vi "AddTemplate.vi"(8 "Error In":errorcluster, 10 "Template-VI Names":string[](array[string])) -> (0 "Error Out":errorcluster)   [LabVIEW 2016]
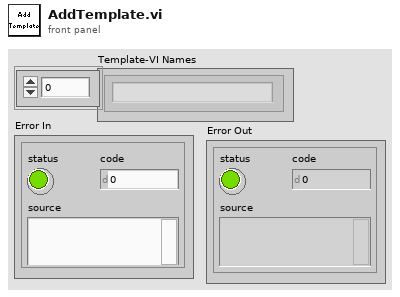
[diagram p1: front panel]
types:
  T1 = enum16{"Invalid Wire Rule", "Required", "Recommended", "Optional", "Dynamic Dispatch"}
  T2 = typedef "LVRectTypeDef.ctl" = cluster{"Left":i16, "Top":i16, "Right":i16, "Bottom":i16}
  T3 = enum16{"Invalid Wire Rule", "Required", "Recommended", "Optional", "Dynamic Dispatch"}[]
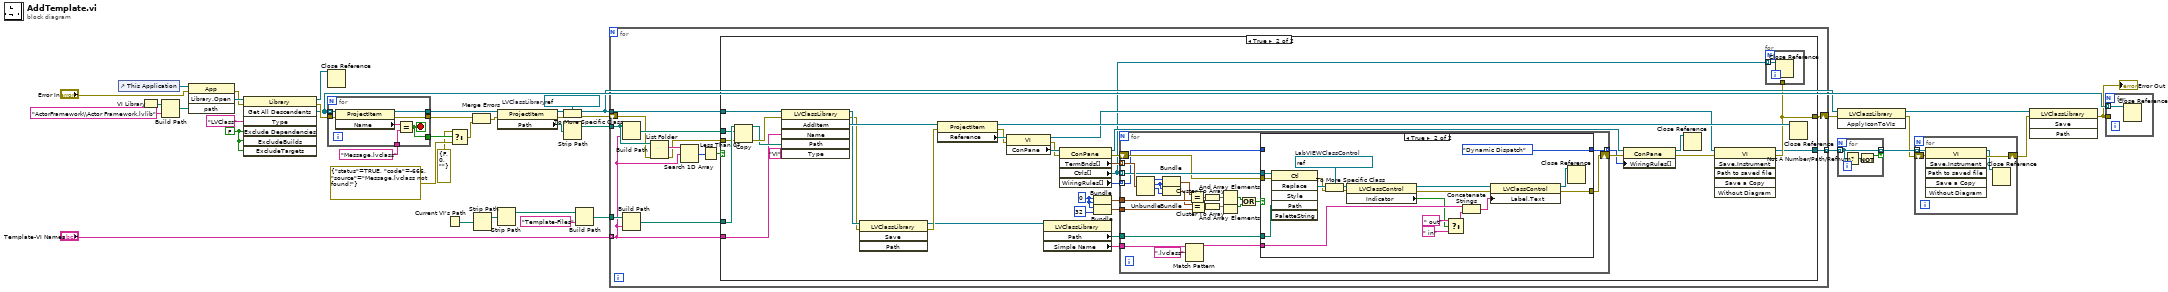
[diagram p0: block diagram]
diagram:
  w18 = refnum<vi> refnum  # LVClassLibrary
  w33 = FALSE ("ExcludeDependencies")
  n1 = control-ref of="This Application"() -> (w40:refnum<vi>)
  n2 = VI Library() -> (path=w39:path)
  n3 = Build Path(base path=w39, name or relative path="ActorFramework\\Actor Framework.lvlib") -> (appended path=w37:path)
  n4 = invoke class="App" method="Library.Open"(reference=w40, error in="Error In", "path"=w37) -> (error out=w34:errorcluster, "Open Library"=w35:refnum<vi>)  [unwired: 1 in, 2 out]
  n5 = invoke class="Library" method="Get All Descendents"(reference=w35, error in=w34, "Type"="LVClass", "Exclude Dependencies"=w33, "ExcludeBuilds"=w33, "ExcludeTargets"=w33) -> (reference out=w6:refnum<vi>, error out=w32:errorcluster, "All Descendents"=w15:refnum<vi>[])  [unwired: 1 in, 4 out]
  n6 = Close Reference(reference=w6) -> ()  [unwired: 1 in, 1 out]
  n7 = for {
    tunnel: w15 -> [w47] mode=indexing
    tunnel: "Message.lvclass" ("name") -> [w45]
    tunnel: [w44] -> w21
    tunnel: w32 -> [w43]
    tunnel: [w42] -> w26
    tunnel: [w41] -> w30
    stop <- w41 stop-if-true
    n8 = property class="ProjectItem"(reference=w47, error in=w43) -> (reference out=w44:refnum<vi>, error out=w42:errorcluster, "Name"=w46:string)
    n9 = Equal?(x=w46, y=w45) -> (x = y?=w41:bool)
  }
  n10 = Current VI's Path() -> (path=w25:path)
  n11 = Select(t=errorcluster {"status"=FALSE, "code"=0, "source"=""} ("error constant"), s=w30, f=errorcluster {"status"=TRUE, "code"=-666, "source"="Message.lvclass not found!"} ("error constant")) -> (s? t:f=w27:errorcluster)
  n12 = Merge Errors(w26, w27) -> (w20:errorcluster)
  n13 = Strip Path(path=w25) -> (stripped path=w24:path)  [unwired: 1 out]
  n14 = Strip Path(path=w24) -> (stripped path=w11:path)  [unwired: 1 out]
  n15 = property class="ProjectItem"(reference=w21, error in=w20) -> (reference out=w17:refnum<vi>, error out=w16:errorcluster, "Path"=w19:path)
  n16 = To More Specific Class(target class=w18, reference=w17, error in=w16) -> (specific class reference=w5:refnum<vi>, error out=w13:errorcluster)
  n17 = Strip Path(path=w19) -> (stripped path=w14:path)  [unwired: 1 out]
  n18 = Build Path(base path=w11, name or relative path="Template-Files") -> (appended path=w22:path)
  n19 = for {
    tunnel: w22 -> [w60]
    tunnel: w5 -> [w58]
    tunnel: w14 -> [w56]
    tunnel: "Template-VI Names" -> [w49] mode=indexing
    shift-right: [w50] -> w8
    shift-left: w13 -> [w55]
    tunnel: [w48] -> w4 mode=indexing
    n20 = Build Path(base path=w56, name or relative path=w49) -> (appended path=w57:path)
    n21 = Build Path(base path=w60, name or relative path=w49) -> (appended path=w59:path)
    n22 = List Folder(path=w56, error in=w55) -> (filenames=w54:string[], error out=w53:errorcluster)  [unwired: 2 in, 2 out]
    n23 = Search 1D Array(1D array=w54, element=w49) -> (index of element=w52:i32)  [unwired: 1 in]
    n24 = Less Than 0?(x=w52) -> (x < 0?=w51:bool)
    n25 = case shown="True" w51 {
      tunnel: w59 -> [_ w93]
      tunnel: w58 -> [_ w91]
      tunnel: [w61 w66] -> w50
      tunnel: w57 -> [_ w65]
      tunnel: w53 -> [w61 w64]
      tunnel: w49 -> [_ w63]
      tunnel: [_ w62] -> w48
      frame False {
      }
      frame True {
        w79 = i16 0
        n26 = Copy(8:w64, 10:w65, 11:w93) -> (0:w94:errorcluster, 3:w92:path)  [unwired: 2 in, 1 out]
        n27 = invoke class="LVClassLibrary" method="AddItem"(reference=w91, error in=w94, "Name"=w63, "Path"=w92, "Type"="VI") -> (reference out=w90:refnum<vi>, error out=w89:errorcluster, "AddItem"=w96:refnum<vi>)  [unwired: 1 in, 3 out]
        n28 = invoke class="LVClassLibrary" method="Save"(reference=w90, error in=w89) -> (reference out=w71:refnum<vi>, error out=w88:errorcluster)  [unwired: 2 in, 2 out]
        n29 = property class="ProjectItem"(reference=w96, error in=w88) -> (reference out=w95:refnum<vi>, error out=w72:errorcluster, "Reference"=w73:refnum<vi>)
        n30 = property class="VI"(reference=w73, error in=w72) -> (reference out=w70:refnum<vi>, error out=w86:errorcluster, "ConPane"=w87:refnum<vi>)
        n31 = property class="LVClassLibrary"(reference=w71) -> ("Path"=w80:path, "Simple Name"=w74:string)  [unwired: 1 in, 2 out]
        n32 = property class="ConPane"(reference=w87, error in=w86) -> (reference out=w76:refnum<vi>, error out=w84:errorcluster, "TermBnds[]"=w85:T2[], "Ctrls[]"=w67:refnum<vi>[], "WiringRules[]"=w78:T3)
        n33 = Bundle(w79, w79) -> (w82:cluster{i16, i16})  [unwired: 1 in]
        n34 = Bundle(w79, i16 32) -> (w81:cluster{i16, i16})  [unwired: 1 in]
        n35 = for {
          tunnel: w85 -> [w121] mode=indexing
          tunnel: w67 -> [w111] mode=indexing
          shift-right: [w105] -> w77
          shift-left: w84 -> [w110]
          tunnel: w82 -> [w118]
          tunnel: w81 -> [w116]
          tunnel: w80 -> [w106]
          tunnel: w78 -> [w102] mode=indexing
          tunnel: [w101] -> w75 mode=indexing
          tunnel: w74 -> [w100]
          n36 = Unbundle(w121) -> ("Left"=w120:i16, "Top"=w103:i16, "Right"=w104:i16)  [unwired: 1 out]
          n37 = Bundle("Left"=w120, "Top"=w103) -> (w119:cluster{"Left":i16, "Top":i16})  [unwired: 1 in]
          n38 = Bundle("Top"=w103, "Right"=w104) -> (w117:cluster{"Top":i16, "Right":i16})  [unwired: 1 in]
          n39 = Match Pattern(string=w100, regular expression=".lvclass") -> (before substring=w99:string)  [unwired: 1 in, 3 out]
          n40 = Equal?(x=w119, y=w118) -> (x = y?=w115:cluster{bool, bool})
          n41 = Equal?(x=w117, y=w116) -> (x = y?=w114:cluster{bool, bool})
          n42 = Cluster To Array(cluster=w115) -> (array=w113:bool[])
          n43 = Cluster To Array(cluster=w114) -> (array=w112:bool[])
          n44 = And Array Elements(Boolean array=w113) -> (logical AND=w109:bool)
          n45 = And Array Elements(Boolean array=w112) -> (logical AND=w108:bool)
          n46 = Or(x=w109, y=w108) -> (x .or. y?=w107:bool)
          n47 = case shown="True" w107 {
            tunnel: w111 -> [_ w142]
            tunnel: w110 -> [w123 w141]
            tunnel: [w123 w137] -> w105
            tunnel: w106 -> [_ w140]
            tunnel: w102 -> [w122 _]
            tunnel: [w122 T1."Dynamic Dispatch" ("Wire Rule")] -> w101
            tunnel: w99 -> [_ w135]
            frame False {
            }
            frame True {
              w138 = refnum<vi> refnum  # LabVIEWClassControl
              n48 = invoke class="Ctl" method="Replace"(reference=w142, error in=w141, "Path"=w140) -> (error out=w129:errorcluster, "Replace"=w130:refnum<vi>)  [unwired: 3 in, 4 out]
              n49 = To More Specific Class(target class=w138, reference=w130, error in=w129) -> (specific class reference=w128:refnum<vi>, error out=w125:errorcluster)
              n50 = property class="LVClassControl"(reference=w128, error in=w125) -> (reference out=w127:refnum<vi>, error out=w126:errorcluster, "Indicator"=w124:bool)
              n51 = Select(t=" out", s=w124, f=" in") -> (s? t:f=w133:string)
              n52 = Concatenate Strings(w135, w133) -> (w134:string)
              n53 = property class="LVClassControl"(reference=w127, error in=w126, "Label.Text"=w134) -> (reference out=w136:refnum<vi>, error out=w137:errorcluster)
              n54 = Close Reference(reference=w136) -> ()  [unwired: 1 in, 1 out]
            }
          }
        }
        n55 = property class="ConPane"(reference=w76, error in=w77, "WiringRules[]"=w75) -> (reference out=w68:refnum<vi>, error out=w69:errorcluster)
        n56 = Close Reference(reference=w68) -> ()  [unwired: 1 in, 1 out]
        n57 = invoke class="VI" method="Save.Instrument"(reference=w70, error in=w69) -> (reference out=w62:refnum<vi>, error out=w66:errorcluster)  [unwired: 4 in, 4 out]
        n58 = for {
          tunnel: w67 -> [w143] mode=indexing
          tunnel: w66 -> [_]
          n59 = Close Reference(reference=w143) -> ()  [unwired: 1 in, 1 out]
        }
        n60 = Close Reference(reference=w95) -> ()  [unwired: 1 in, 1 out]
      }
    }
  }
  n61 = invoke class="LVClassLibrary" method="ApplyIconToVIs"(reference=w5, error in=w8) -> (reference out=w9:refnum<vi>, error out=w2:errorcluster)  [unwired: 1 in, 1 out]
  n62 = for {
    tunnel: w4 -> [w146] mode=indexing
    tunnel: [w146] -> w3 mode=indexing if=w144
    n63 = Not A Number/Path/Refnum?(number/path/refnum=w146) -> (NaN/Path/Refnum?=w145:bool)
    n64 = Not(x=w145) -> (.not. x?=w144:bool)
  }
  n65 = for {
    tunnel: w3 -> [w150] mode=indexing
    shift-right: [w148] -> w1
    shift-left: w2 -> [w149]
    n66 = invoke class="VI" method="Save.Instrument"(reference=w150, error in=w149) -> (reference out=w147:refnum<vi>, error out=w148:errorcluster)  [unwired: 4 in, 4 out]
    n67 = Close Reference(reference=w147) -> ()  [unwired: 1 in, 1 out]
  }
  n68 = invoke class="LVClassLibrary" method="Save"(reference=w9, error in=w1) -> (error out=w7:errorcluster)  [unwired: 2 in, 3 out]
  "Error Out" <- w7
  n69 = for {
    tunnel: w7 -> [_]
    tunnel: w15 -> [w151] mode=indexing
    n70 = Close Reference(reference=w151) -> ()  [unwired: 1 in, 1 out]
  }
